vi "sub_setpos_fgv.vi"(7 "cmd":enum16{"read", "init", "left", "write", "right"}(ring), 11 "Slide":dbl(slide) scale=-1.0..1.0) -> (2 "out_range":bool, 3 "set_pos":dbl)   [LabVIEW 2018]
uses:
  Global_val.vi
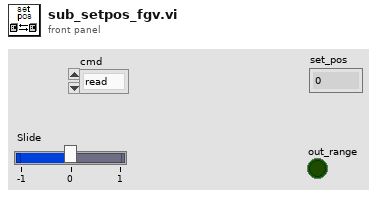
[diagram p1: front panel]
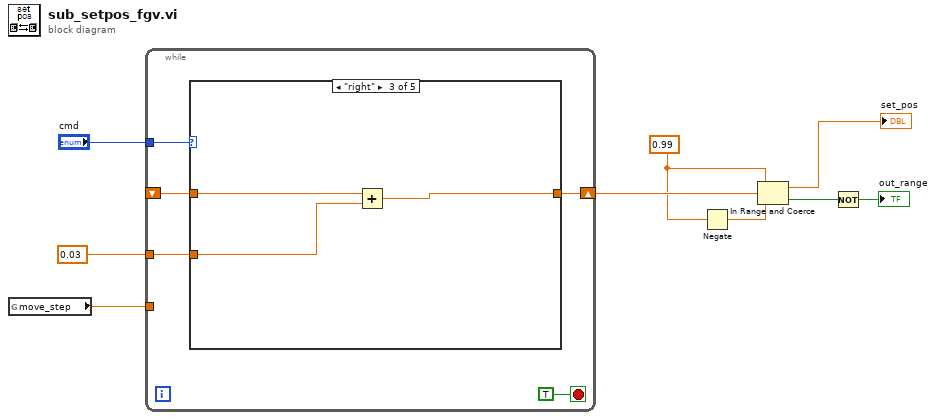
[diagram p0: block diagram]
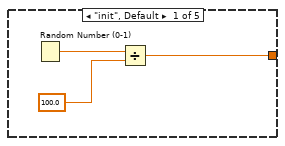
[diagram p2: hidden frame]
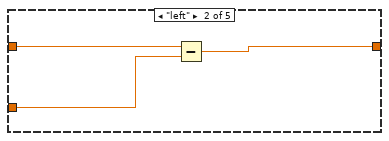
[diagram p3: hidden frame]
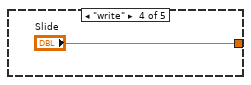
[diagram p4: hidden frame]
diagram:
  w7 = 0.99
  n1 = global read "Global_val.vi" "move_step"() -> (w1:dbl)
  n2 = while {
    tunnel: "cmd" -> [w13]
    shift-right: [w12] -> w8
    shift-left: _ -> [w11]
    tunnel: 0.03 -> [w10]
    tunnel: w1 -> [_]
    stop <- TRUE stop-if-true
    n3 = case shown="\"right\"" w13 {
      tunnel: [w15 w18 w21 "Slide" w25] -> w12
      tunnel: w11 -> [_ w20 w23 _ w25]
      tunnel: w10 -> [_ w19 w22 _ _]
      frame "init", Default {
        n4 = Random Number (0-1)() -> (number: 0 to 1=w17:dbl)
        n5 = Divide(x=w17, y=100.0) -> (x/y=w15:dbl)
      }
      frame "left" {
        n6 = Subtract(x=w20, y=w19) -> (x-y=w18:dbl)
      }
      frame "right" {
        n7 = Add(x=w23, y=w22) -> (x+y=w21:dbl)
      }
      frame "write" {
      }
      frame "read" {
      }
    }
  }
  n8 = Negate(x=w7) -> (-x=w6:dbl)
  n9 = In Range and Coerce(upper limit=w7, x=w8, lower limit=w6) -> (coerced(x)=→"set_pos":dbl, In Range?=w4:bool)
  n10 = Not(x=w4) -> (.not. x?=→"out_range":bool)
